vi "Test VI.vi"(8 "error in (no error)":errorcluster, 10 "Project Path":path=path "E:/sw-deps-monitor/Source/BuildSpecs/Modules/ModuleA.lvproj") -> (0 "error out":errorcluster)   [LabVIEW 2019, in "Hawkeye.lvlib"]
uses:
  Hawkeye.lvlib
panel:
  in  "Project Ref":refnum<vi>
  in  "reference":refnum<vi>
  out "Claimed Class":path[](array[path])
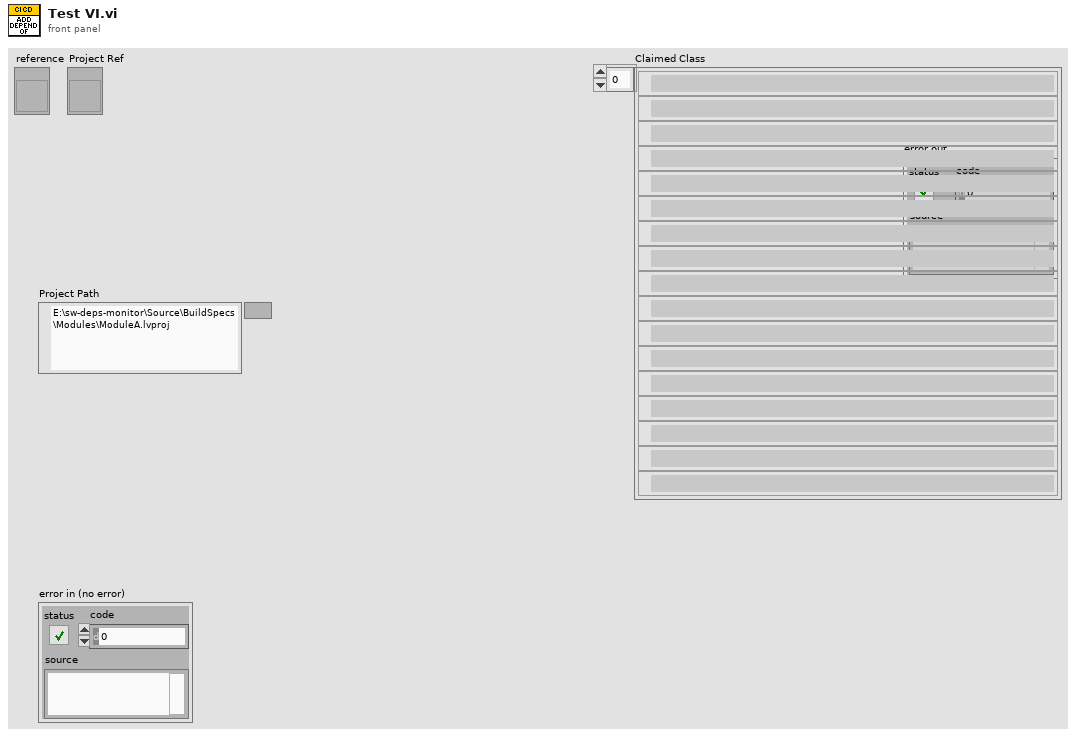
[diagram p1: front panel]
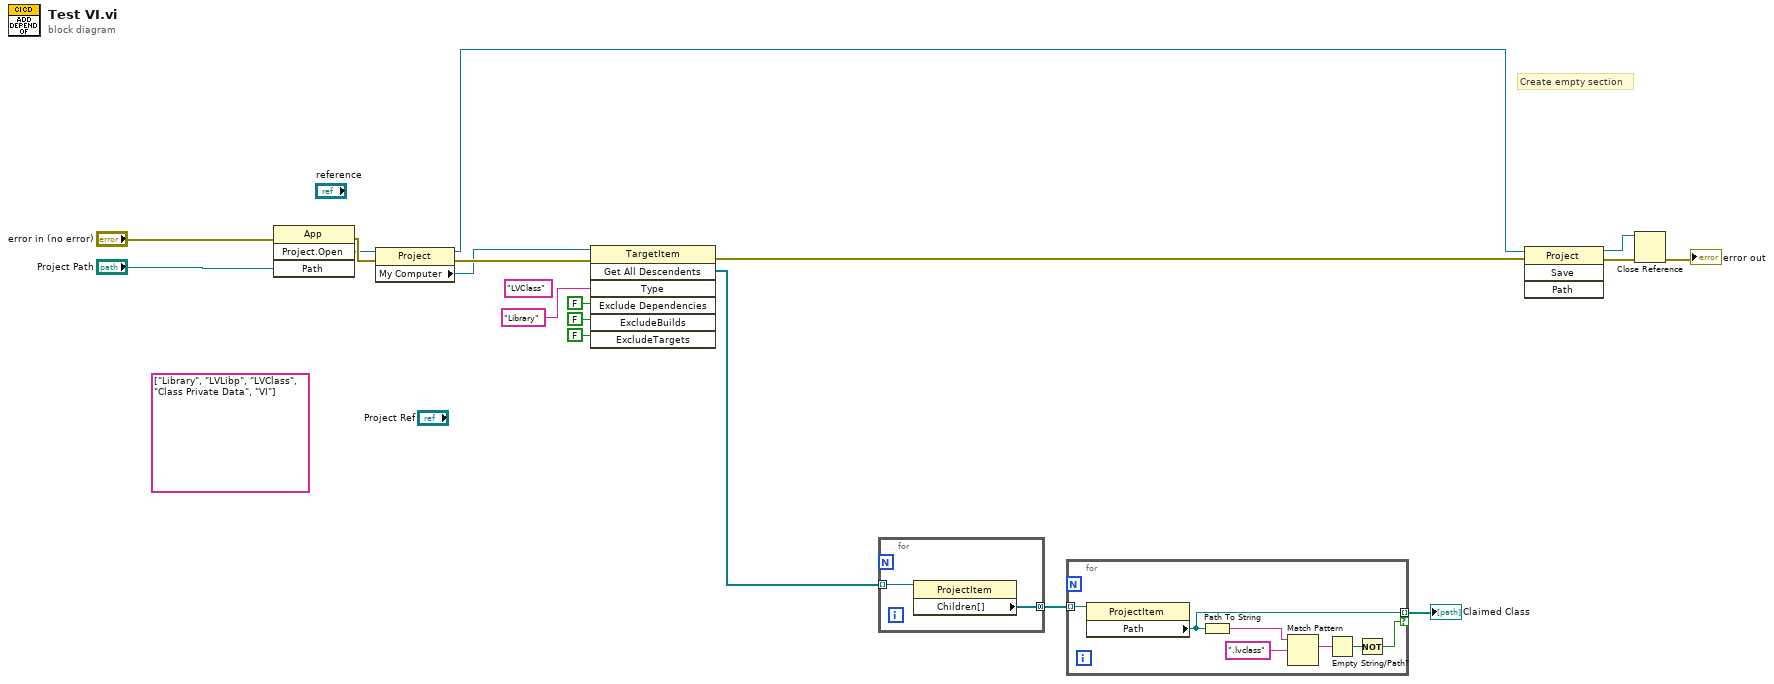
[diagram p0: block diagram]
diagram:
  (unwired) "LVClass" ("Type")
  (unwired) string[] ["Library", "LVLibp", "LVClass", "Class Private Data", "VI"] ("Type")
  # "Create empty section"
  n1 = invoke class="App" method="Project.Open"(error in="error in (no error)", "Path"="Project Path") -> (error out=w17:errorcluster, "Project:Open"=w6:refnum<vi>)  [unwired: 2 in, 2 out]
  n2 = property class="Project"(reference=w6, error in=w17) -> (reference out=w11:refnum<vi>, error out=w13:errorcluster, "My Computer"=w5:refnum<vi>)
  n3 = invoke class="TargetItem" method="Get All Descendents"(reference=w5, error in=w13, "Type"="Library", "Exclude Dependencies"=FALSE ("ExcludeDependencies"), "ExcludeBuilds"=FALSE, "ExcludeTargets"=FALSE) -> (error out=w12:errorcluster, "All Descendents"=w4:refnum<vi>[])  [unwired: 1 in, 5 out]
  n4 = for {
    tunnel: w4 -> [w20] mode=indexing
    tunnel: [w19] -> w2 mode=concatenating
    n5 = property class="ProjectItem"(reference=w20) -> ("Children[]"=w19:refnum<vi>[])  [unwired: 1 in, 2 out]
  }
  n6 = for {
    tunnel: w2 -> [w27] mode=indexing
    tunnel: [w23] -> w1 mode=indexing if=w21
    n7 = property class="ProjectItem"(reference=w27) -> ("Path"=w23:path)  [unwired: 1 in, 2 out]
    n8 = Path To String(path=w23) -> (string=w26:string)
    n9 = Match Pattern(string=w26, regular expression=".lvclass") -> (match substring=w24:string)  [unwired: 1 in, 3 out]
    n10 = Empty String/Path?(string/path=w24) -> (empty?=w22:bool)
    n11 = Not(x=w22) -> (.not. x?=w21:bool)
  }
  "Claimed Class" <- w1
  n12 = invoke class="Project" method="Save"(reference=w11, error in=w12) -> (reference out=w10:refnum<vi>, error out=w9:errorcluster)  [unwired: 2 in, 2 out]
  n13 = Close Reference(reference=w10, error in (no error)=w9) -> (error out=→"error out":errorcluster)
